vi "RT fifos.vi"   [LabVIEW 2019]
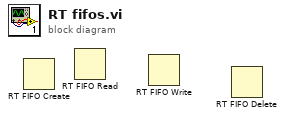
[diagram p0: block diagram]
diagram:
  n1 = RT FIFO Create() -> ()  [unwired: 8 in, 3 out]
  n2 = RT FIFO Read() -> ()  [unwired: 4 in, 5 out]
  n3 = RT FIFO Write() -> ()  [unwired: 5 in, 4 out]
  n4 = RT FIFO Delete() -> ()  [unwired: 3 in, 1 out]
